vi "BGA244_get.vi"(8 "error in":errorcluster, 10 "string in":string, 11 "VISA in":refnum<visa-resource-name>) -> (0 "error out":errorcluster, 2 "string out":string, 3 "VISA out":refnum<visa-resource-name>)   [LabVIEW 2019]
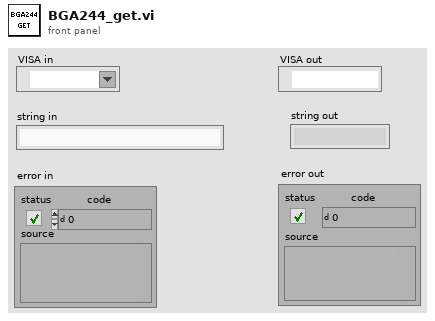
[diagram p1: front panel]
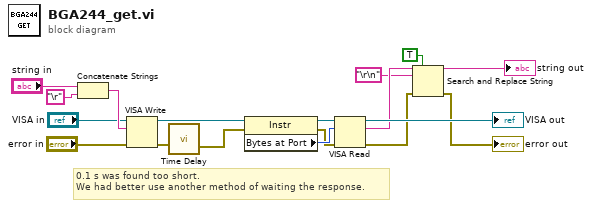
[diagram p0: block diagram]
diagram:
  # "0.1 s was found too short.\nWe had better use another method of waiting the response."
  n1 = Concatenate Strings("string in", "\r") -> (w15:string)
  n2 = VISA Write(VISA resource name="VISA in", write buffer=w15, error in (no error)="error in") -> (VISA resource name out=w18:refnum<visa-resource-name>, error out=w11:errorcluster)  [unwired: 1 out]
  n3 = call "Time Delay"("error in (no error)"=w11) -> ("error out"=w10:errorcluster)  [unwired: 10 in]
  n4 = property class="Instr"(reference=w18, error in=w10) -> (reference out=w17:refnum<visa-resource-name>, error out=w12:errorcluster, "Bytes at Port"=w14:u32)
  n5 = VISA Read(VISA resource name=w17, byte count=w14, error in (no error)=w12) -> (VISA resource name out=→"VISA out":refnum<visa-resource-name>, read buffer=w6:string, error out=w4:errorcluster)  [unwired: 1 out]
  n6 = Search and Replace String(replace all?=TRUE ("replace all? (F)"), input string=w6, search string="\r\n", error in=w4) -> (result string=→"string out":string, error out=→"error out":errorcluster)  [unwired: 4 in, 2 out]
